vi "BRig_dataMTrig_Audio_N_L.vi"() -> (2 "output_Audio_N_L":i32)   [LabVIEW 2014]
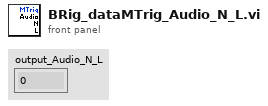
[diagram p1: front panel]
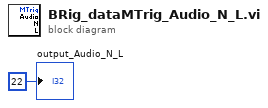
[diagram p0: block diagram]
diagram:
  "output_Audio_N_L" <- 22 ("output_iBlock")
